vi "matriz-1D.vi"() -> ()   [LabVIEW 2020]
panel:
  out "Numeric":dbl
  out "Array":dbl[](array[numeric])
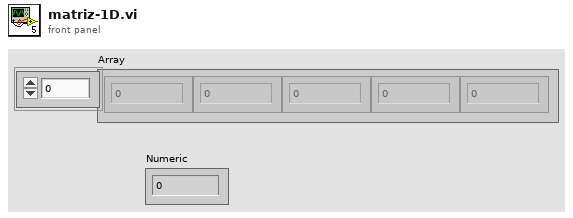
[diagram p1: front panel]
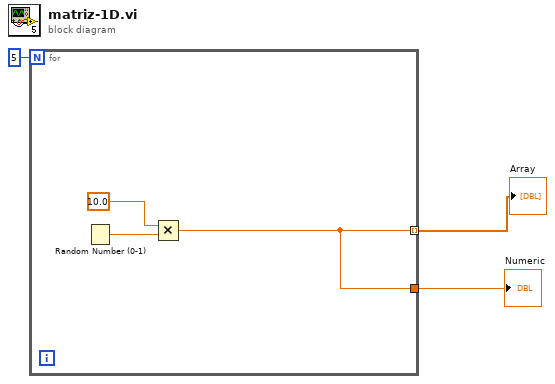
[diagram p0: block diagram]
diagram:
  n1 = for {
    N: 5 -> [_]
    tunnel: [w4] -> w2 mode=indexing
    tunnel: [w4] -> w1
    n2 = Random Number (0-1)() -> (number: 0 to 1=w6:dbl)
    n3 = Multiply(x=10.0, y=w6) -> (x*y=w4:dbl)
  }
  "Array" <- w2
  "Numeric" <- w1
